vi "test.vi"() -> ()   [LabVIEW 2014]
uses:
  <vilib>/measure/matone.llb/Extract Single Tone Information N Chan.vi
  <vilib>/measure/NI_MAPro.lvlib
panel:
  in  "Example tone":path
  in  "Play Example Tone(The target tone which is expected result from the averaged tone1&2)":bool
  in  "Play Mixed Tone 1 & Tone 2":bool
  out "Tone 2 waveform":waveform(dbl)[](graph)
  in  "Play Mergerd Tone1&Tone2":bool
  out "Tone 1 waveform":waveform(dbl)[](graph)
  out "Merged Wavefrom":dynamicdata(graph)
  in  "Tone2":path
  in  "Tone1":path
  in  "Play Tone2":bool
  in  "Play Tone1":bool
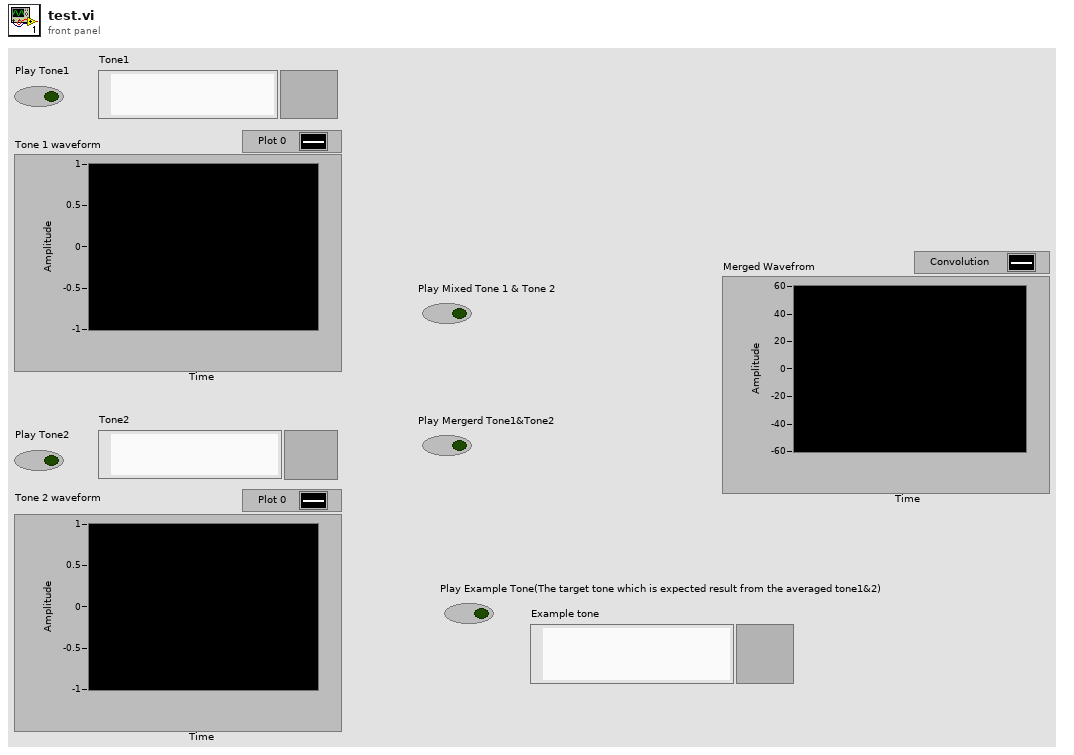
[diagram p1: front panel]
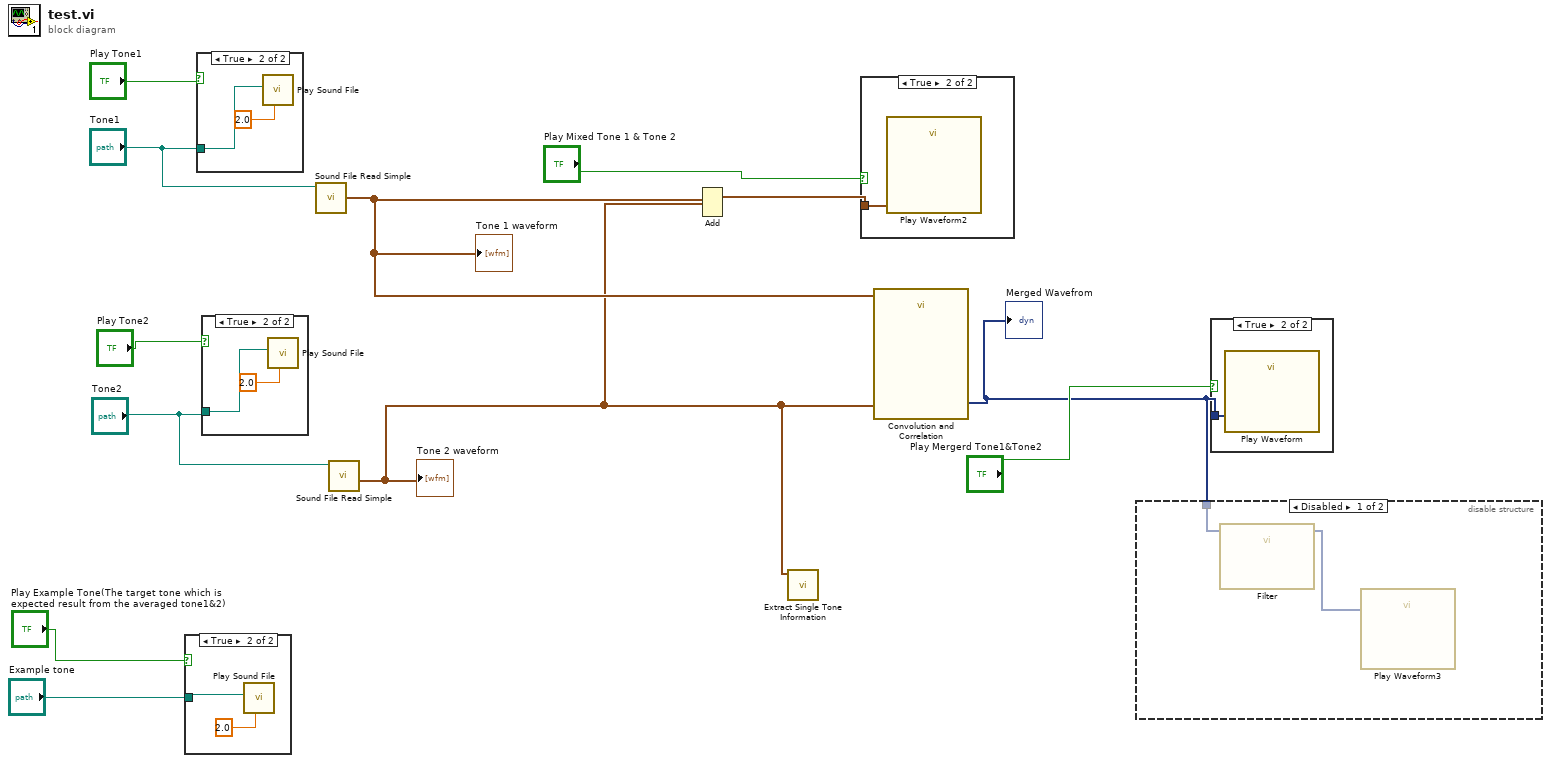
[diagram p0: block diagram]
diagram:
  n1 = case shown="True" "Play Example Tone(The target tone which is expected result from the averaged tone1&2)" {
    tunnel: "Example tone" -> [_ w13]
    frame False {
    }
    frame True {
      n2 = call <vilib>:"Play Sound File.vi"("timeout (sec)"=2.0, "path"=w13) -> ()  [unwired: 8 in, 2 out]
    }
  }
  n3 = case shown="True" "Play Tone1" {
    tunnel: "Tone1" -> [_ w15]
    frame False {
    }
    frame True {
      n4 = call <vilib>:"Play Sound File.vi"("timeout (sec)"=2.0, "path"=w15) -> ()  [unwired: 8 in, 2 out]
    }
  }
  n5 = case shown="True" "Play Tone2" {
    tunnel: "Tone2" -> [_ w17]
    frame False {
    }
    frame True {
      n6 = call <vilib>:"Play Sound File.vi"("timeout (sec)"=2.0, "path"=w17) -> ()  [unwired: 8 in, 2 out]
    }
  }
  n7 = call <vilib>:"Sound File Read Simple.vi"("path"="Tone1") -> ("data"=w6:waveform(dbl)[])  [unwired: 7 in, 3 out]
  "Tone 1 waveform" <- w6
  n8 = call <vilib>:"Sound File Read Simple.vi"("path"="Tone2") -> ("data"=w1:waveform(dbl)[])  [unwired: 7 in, 3 out]
  "Tone 2 waveform" <- w1
  n9 = Add(1:w1, 2:w6) -> (0:w7:waveform(dbl)[])  [unwired: 1 in, 1 out]
  n10 = call-poly <vilib>:"Extract Single Tone Information.vi"("time signals in"=w1) -> ()  [unwired: 5 in, 6 out]
  n11 = case shown="True" "Play Mixed Tone 1 & Tone 2" {
    tunnel: w7 -> [_ w19]
    frame False {
    }
    frame True {
      n12 = call "Play Waveform2"("Data"=w19) -> ()  [unwired: 18 in, 1 out]
    }
  }
  n13 = call "Convolution and Correlation"("Y"=w1, "X"=w6) -> ("X*Y"=w2:dynamicdata)  [unwired: 8 in, 1 out]
  "Merged Wavefrom" <- w2
  n14 = disable-structure shown="Disabled" {
    disable-tunnel: w2 -> [w21 _]
    frame Disabled {
      n15 = call "Filter"("Signal"=w21) -> ("Filtered Signal"=w20:dynamicdata)  [unwired: 9 in, 1 out]
      n16 = call "Play Waveform3"("Data"=w20) -> ()  [unwired: 18 in, 1 out]
    }
    frame Enabled {
    }
  }
  n17 = case shown="True" "Play Mergerd Tone1&Tone2" {
    tunnel: w2 -> [_ w22]
    frame False {
    }
    frame True {
      n18 = call "Play Waveform"("Data"=w22) -> ()  [unwired: 18 in, 1 out]
    }
  }
